vi "Read Int_limit.vi"(8 "error in (no error)":errorcluster, 11 "Non Linear PID Controller in":refnum<class "Non Linear PID Controller.lvclass">) -> (0 "error out":errorcluster, 2 "Int_limit":dbl[](array[numeric]), 3 "Non Linear PID Controller out":refnum<class "Non Linear PID Controller.lvclass">)   [LabVIEW 2014, in "Controller Library.lvlib" / "Non Linear PID Controller.lvclass"]
uses:
  Non Linear PID Controller.lvclass
  Non Linear PID Controller.lvclass/Non Linear PID Controller.ctl
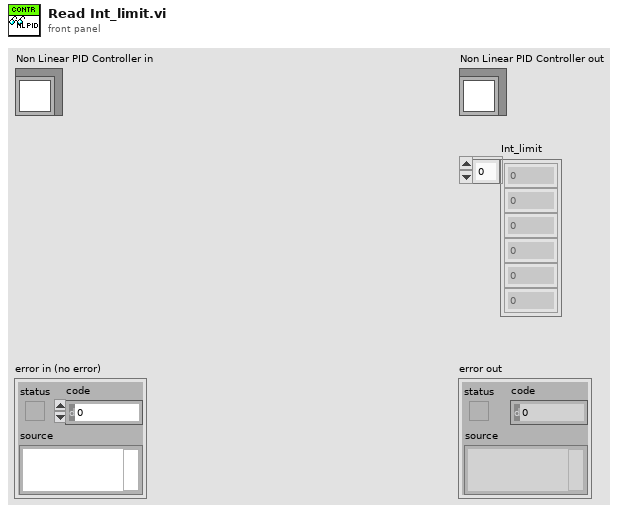
[diagram p1: front panel]
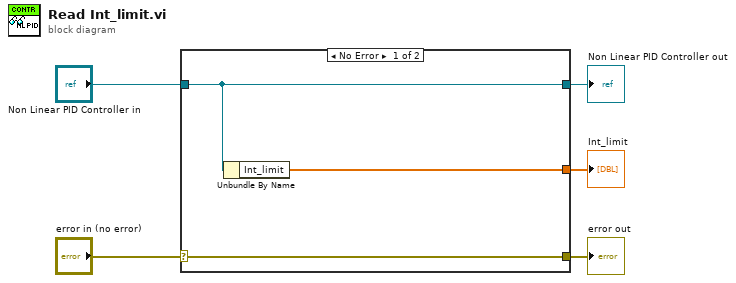
[diagram p0: block diagram]
diagram:
  n1 = case shown="No Error" "error in (no error)" {
    selector: "error in (no error)" -> [w8 w9]
    tunnel: [w8 w9] -> w4
    tunnel: [w7 w10] -> w2
    tunnel: "Non Linear PID Controller in" -> [w7 w10]
    tunnel: [w6 _] -> w1
    frame No Error {
      n2 = Unbundle By Name(w7) -> ("Int_limit"=w6:dbl[])
    }
    frame Error {
    }
  }
  "error out" <- w4
  "Non Linear PID Controller out" <- w2
  "Int_limit" <- w1
